vi "Read Gluing Parameters.vi"(8 "error in (no error)":errorcluster, 11 "Config Manager Class in":refnum<class "Config Manager Class.lvclass">) -> (0 "error out":errorcluster, 2 "Gluing Parameters":T1, 3 "Config Manager Class out":refnum<class "Config Manager Class.lvclass">)   [LabVIEW 2011, in "Config Manager Class.lvclass"]
uses:
  Config Manager Class.lvclass
  Type Definitions/Gluing Parameters.ctl
  Config Manager Class.lvclass/Config Manager Class.ctl
  <vilib>/Utility/config.llb/Read Key (Double).vi
  <vilib>/Utility/config.llb/NI_LVConfig.lvlib
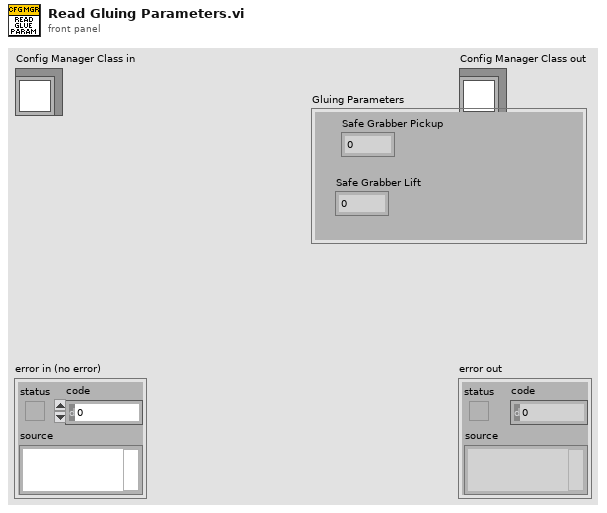
[diagram p1: front panel]
types:
  T1 = typedef "Gluing Parameters.ctl" = cluster{"Safe Grabber Pickup":dbl, "Safe Grabber Lift":dbl}
  T2 = typedef "NI_LVConfig.lvlib/Config Data RefNum.ctl" = refnum<k1>
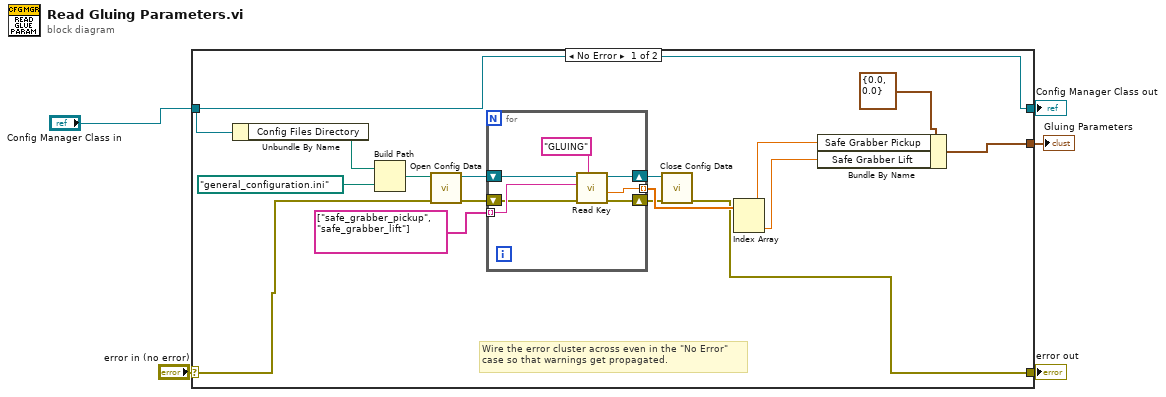
[diagram p0: block diagram]
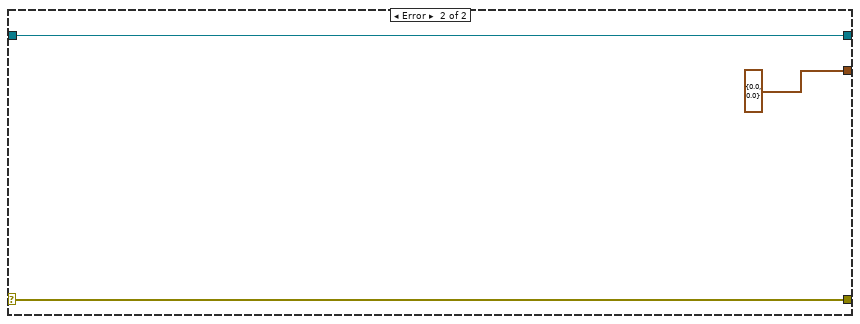
[diagram p2: hidden frame]
diagram:
  n1 = case shown="No Error" "error in (no error)" {
    selector: "error in (no error)" -> [w12 w31]
    tunnel: "Config Manager Class in" -> [w8 w30]
    tunnel: [w8 w30] -> w3
    tunnel: [w9 T1 {"Safe Grabber Pickup"=0.0, "Safe Grabber Lift"=0.0} ("Gluing Parameters 2")] -> w2
    tunnel: [w7 w31] -> w1
    frame No Error {
      # "Wire the error cluster across even in the \"No Error\"\ncase so that warnings get propagated."
      n2 = Unbundle By Name(w8) -> ("Config Files Directory"=w15:path)
      n3 = Build Path(base path=w15, name or relative path=path "general_configuration.ini") -> (appended path=w14:path)
      n4 = call <vilib>:"Open Config Data.vi"("error in (no error)"=w12, "configuration file path"=w14) -> ("error out"=w18:errorcluster, "refnum"=w17:T2)  [unwired: 7 in, 1 out]
      n5 = for {
        tunnel: string[] ["safe_grabber_pickup", "safe_grabber_lift"] -> [w25] mode=indexing
        shift-right: [w26] -> w20
        shift-left: w17 -> [w27]
        tunnel: [w23] -> w21 mode=indexing
        shift-right: [w22] -> w19
        shift-left: w18 -> [w24]
        n6 = call-poly <vilib>:"Read Key.vi"("section"="GLUING", "error in (no error)"=w24, "key"=w25, "refnum"=w27) -> ("error out"=w22:errorcluster, "value"=w23:dbl, "refnum out"=w26:T2)  [unwired: 4 in, 1 out]
      }
      n7 = call <vilib>:"Close Config Data.vi"("error in (no error)"=w19, "refnum"=w20) -> ("error out"=w7:errorcluster)  [unwired: 8 in, 1 out]
      n8 = Index Array(array=w21) -> (element #1=w11:dbl, element #2=w6:dbl)  [unwired: 2 in]
      n9 = Bundle By Name(cluster=T1 {"Safe Grabber Pickup"=0.0, "Safe Grabber Lift"=0.0} ("Gluing Parameters"), "Safe Grabber Pickup"=w11, "Safe Grabber Lift"=w6) -> (w9:T1)
    }
    frame Error {
    }
  }
  "error out" <- w1
  "Config Manager Class out" <- w3
  "Gluing Parameters" <- w2
